vi "Layout.vi"(8 "ErrorIn":errorcluster, 11 "ReferenceIn":refnum<class "MasterGUI.lvclass">) -> (0 "ErrorOut":errorcluster, 3 "ReferenceIn":refnum<class "MasterGUI.lvclass">)   [LabVIEW 2021, in "MasterGUI.lvclass"]
uses:
  MasterGUI.lvclass
  c12fd466-6d7f-429f-8d31-7d2924c23ef2.vi
  <vilib>/Utility/Data Type/Get Cluster Information.vi
  <vilib>/Utility/Data Type/Get Type Information.vi
  MasterGUI.lvclass/MasterGUI.ctl
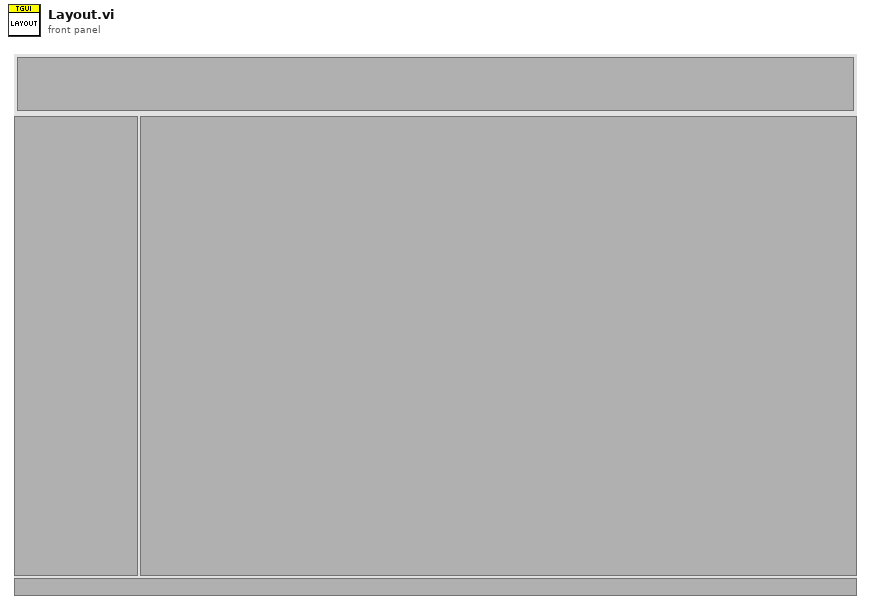
[diagram p1: front panel]
types:
  T1 = cluster{"Header":refnum<vi>, "ButtonBar":refnum<vi>, "MainFlexPanel":refnum<vi>, "Footer":refnum<vi>}
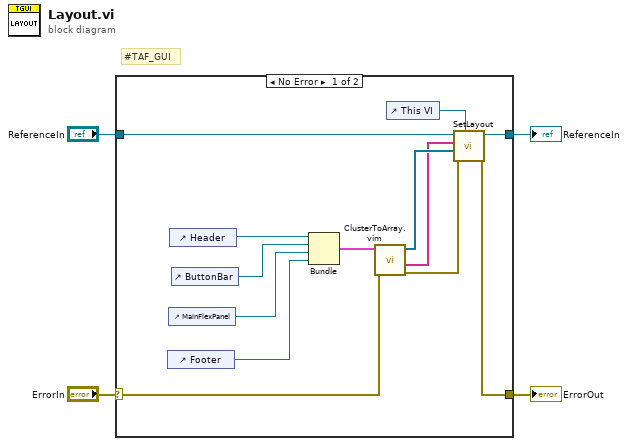
[diagram p0: block diagram]
diagram:
  # "#TAF_GUI"
  n1 = case shown="No Error" "ErrorIn" {
    selector: "ErrorIn" -> [w17 w19]
    tunnel: [w15 w19] -> w3
    tunnel: [w9 w18] -> w1
    tunnel: "ReferenceIn" -> [w8 w18]
    frame No Error {
      n2 = control-ref of="Footer"() -> (w13:refnum<vi>)
      n3 = control-ref of="MainFlexPanel"() -> (w12:refnum<vi>)
      n4 = control-ref of="Header"() -> (w10:refnum<vi>)
      n5 = control-ref of="ButtonBar"() -> (w11:refnum<vi>)
      n6 = Bundle("Header"=w10, "ButtonBar"=w11, "MainFlexPanel"=w12, "Footer"=w13) -> (w14:T1)  [unwired: 1 in]
      n7 = call "ClusterToArray.vim"("ErrorIn"=w17, "Cluster"=w14) -> ("ErrorOut"=w16:errorcluster, "Labels"=w5:string[], "ArrayOfElements"=w6:refnum<vi>[])  [unwired: 7 in]
      n8 = control-ref of="This VI"() -> (w7:refnum<vi>)
      n9 = call-dynamic "SetLayout.vi"("PanelVIRef"=w7, "ErrorIn"=w16, "SubPanels"=w6, "Labels"=w5, "ReferenceIn"=w8) -> ("ErrorOut"=w15:errorcluster, "ReferenceIn"=w9:refnum<class "MasterGUI.lvclass">)  [unwired: 5 in]
    }
    frame Error {
    }
  }
  "ErrorOut" <- w3
  "ReferenceIn" <- w1
